vi "Edit Line.vi"(8 "error in":errorcluster, 10 "Line Name":string, 11 "References":T1) -> (0 "error out":errorcluster, 2 "change?":bool)   [LabVIEW 2013, in "shared memory editor node.lvclass"]
doc: "This VI edits the properties of a line. It will unlink channels and tags and create new links to channels and tags."
uses:
  shared memory editor node.lvclass
  <vilib>/NI/DCAF/Tag Editor Core/Table API/Table Manager/object ref.ctl
  <vilib>/NI/DCAF/Tag Editor Core/Configuration Editor/Classes/Engine Parent/Engine Parent Editor Node.lvclass
  <vilib>/NI/DCAF/Tag Editor Core/Configuration Editor/Classes/Module editor node/module editor node.lvclass
  module/configuration/shared memory configuration.lvclass
  module/configuration/shared memory configuration.lvclass/shared memory configuration.ctl
  <vilib>/NI/Configuration Framework/serializable configuration/NISE_CEF_serializable configuration.lvclass/NISE_CEF_serializable configuration.ctl
  <vilib>/Utility/LVClass/Get LV Class Name.vi
  <vilib>/NI/Configuration Framework/error generator/NISE_error generator.vi
  <vilib>/NI/Configuration Framework/serializable configuration/NISE_CEF_serializable configuration.lvclass
  <vilib>/NI/DCAF/Tag Editor Core/Table API/Table Manager/Table Manager.lvclass
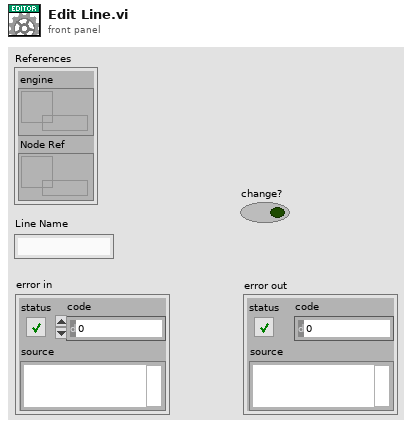
[diagram p1: front panel]
types:
  T1 = typedef "Table Manager.lvlib/Table Manager.lvclass/object ref.ctl" = cluster{"engine":refnum<data-value>, "Node Ref":refnum<data-value>}
  T2 = typedef "shared memory configuration.lvclass/Line.ctl" = cluster{"name":string, "data type":T3, "channel":refnum<class "TBM channel.lvclass">}
  T3 = typedef "tag bus.lvlib/tag descriptor.lvclass/Data Type.ctl" = enum16{"Double", "Single", "I64", "I32", "I16", "I8", "U64", "U32", "U16", "U8", "Boolean", "String", "Array of Double", "Array of Single", "Array of I64", "Array of I32", "Array of I16", "Array of I8", "Array of U64", "Array of U32", "Array of U16", "Array of U8", "Array of Boolean", "Array of String"}
  T4 = typedef "shared memory editor node.lvclass/Mappings.ctl" = cluster{"Line":T2, "Maps":T5[]}
  T5 = typedef "shared memory editor node.lvclass/Map.ctl" = cluster{"channel":refnum<class "TBM channel.lvclass">, "tag name":string}
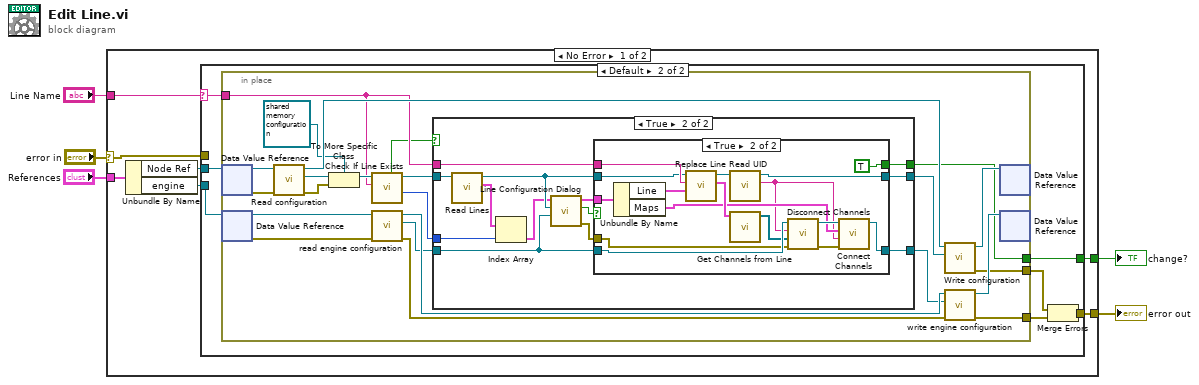
[diagram p0: block diagram]
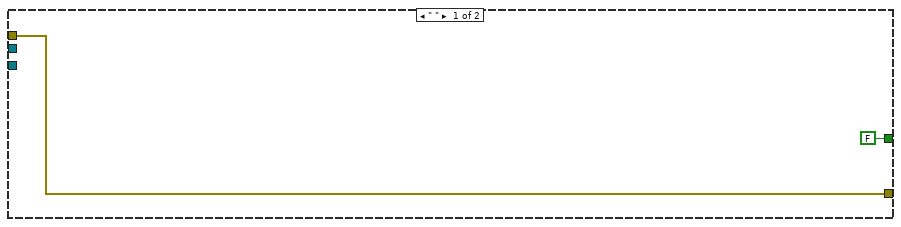
[diagram p2: hidden frame]
diagram:
  n1 = case shown="No Error" "error in" {
    selector: "error in" -> [w6 w78]
    tunnel: "References" -> [w10 _]
    tunnel: "Line Name" -> [w7 _]
    tunnel: [w9 w78] -> w2
    tunnel: [w8 _] -> w1
    frame No Error {
      n2 = Unbundle By Name(w10) -> ("Node Ref"=w12:refnum<data-value>, "engine"=w11:refnum<data-value>)
      n3 = case shown="Default" w7 {
        selector: w7 -> [_ w15]
        tunnel: w12 -> [_ w21]
        tunnel: w11 -> [_ w20]
        tunnel: [w13 w17] -> w9
        tunnel: [FALSE ("change?") w16] -> w8
        tunnel: w6 -> [w13 _]
        frame " " {
        }
        frame Default {
          n4 = in-place {
            in-place-border: [w25] -> w19
            in-place-border: [w41] -> w18
            in-place-border: [w24] -> w16
            in-place-border: w15 -> [w30]
            n5 = in-place-dvr #1(w21) -> (w37:refnum<class "module editor node.lvclass">, w31:errorcluster)
            n6 = in-place-dvr #2(w20) -> (w44:refnum<class "Engine Parent Editor Node.lvclass">, w43:errorcluster)
            n7 = call-dynamic "Read configuration.vi"("error in"=w31, "NISE_CEF_serializable node in"=w37) -> ("error out"=w34:errorcluster, "configuration"=w35:refnum<class "NISE_CEF_serializable configuration.lvclass">, "NISE_CEF_serializable node out"=w36:refnum<class "module editor node.lvclass">)  [unwired: 7 in]
            n8 = To More Specific Class(target class=refnum<class "shared memory configuration.lvclass"> refnum ("tag bus configurable plugin module configuration"), reference=w35, error in=w34) -> (specific class reference=w32:refnum<class "shared memory configuration.lvclass">)  [unwired: 1 out]
            n9 = call-dynamic "Check If Line Exists.vi"("Name to Locate"=w30, "shared memory configuration in"=w32) -> ("Index"=w27:i32, "shared memory configuration out"=w28:refnum<class "shared memory configuration.lvclass">, "Found?"=w22:bool)  [unwired: 5 in, 2 out]
            n10 = call <vilib>:"read engine configuration.vi"("error in"=w43, "Engine Parent Editor Node in"=w44) -> ("error out"=w39:errorcluster, "engine configuration"=w26:refnum<class "engine configuration.lvclass">, "Engine Parent Editor Node out"=w40:refnum<class "Engine Parent Editor Node.lvclass">)  [unwired: 7 in]
            n11 = case shown="True" w22 {
              tunnel: w28 -> [w46 w57]
              tunnel: w26 -> [w45 w47]
              tunnel: w30 -> [_ w59]
              tunnel: [w46 w51] -> w29
              tunnel: w27 -> [_ w54]
              tunnel: [_ w49] -> w24
              tunnel: [w45 w48] -> w23
              frame False {
              }
              frame True {
                n12 = call "Read Lines.vi"("shared memory configuration in"=w57) -> ("Lines"=w55:T2[], "shared memory configuration out"=w56:refnum<class "shared memory configuration.lvclass">)  [unwired: 8 in, 1 out]
                n13 = Index Array(array=w55, index=w54) -> (element=w53:T2)
                n14 = call "Line Configuration Dialog.vi"("engine configuration in"=w47, "tag bus configurable plugin module configuration"=w56, "Line"=w53) -> ("error out"=w58:errorcluster, "changed"=w50:bool, "Mappings out"=w52:T4)  [unwired: 5 in, 1 out]
                n15 = case shown="True" w50 {
                  tunnel: w59 -> [_ w77]
                  tunnel: w47 -> [w60 w76]
                  tunnel: w58 -> [_ w75]
                  tunnel: w56 -> [w61 w71]
                  tunnel: w52 -> [_ w70]
                  tunnel: [w61 w68] -> w51
                  tunnel: [_ TRUE ("change?")] -> w49
                  tunnel: [w60 w62] -> w48
                  frame False {
                  }
                  frame True {
                    n16 = Unbundle By Name(w70) -> ("Line"=w69:T2, "Maps"=w65:T5[])
                    n17 = call "Replace Line.vi"("New Line"=w69, "Line Name"=w77, "shared memory configuration in"=w71) -> ("Old Line"=w73:T2, "shared memory configuration out"=w74:refnum<class "shared memory configuration.lvclass">)  [unwired: 6 in, 1 out]
                    n18 = call <vilib>:"Read UID.vi"("configuration in"=w74) -> ("instance id"=w64:string, "configuration out"=w68:refnum<class "shared memory configuration.lvclass">)  [unwired: 8 in, 1 out]
                    n19 = call "Get Channels from Line.vi"("Line"=w73) -> ("Channels"=w72:refnum<class "TBM channel.lvclass">[])  [unwired: 10 in]
                    n20 = call "Disconnect Channels.vi"("error in (no error)"=w75, "Deleted Channels"=w72, "instance id"=w64, "Engine Configuration in"=w76) -> ("error out"=w66:errorcluster, "Engine Configuration out"=w67:refnum<class "engine configuration.lvclass">)  [unwired: 6 in]
                    n21 = call "Connect Channels.vi"("error in (no error)"=w66, "instance id"=w64, "Maps"=w65, "Engine Configuration in"=w67) -> ("Engine Configuration out"=w62:refnum<class "engine configuration.lvclass">)  [unwired: 6 in, 1 out]
                  }
                }
              }
            }
            n22 = call-dynamic "Write configuration.vi"("configuration"=w29, "NISE_CEF_serializable node in"=w36) -> ("error out"=w25:errorcluster, "NISE_CEF_serializable node out"=w38:refnum<class "module editor node.lvclass">)  [unwired: 8 in]
            n23 = call <vilib>:"write engine configuration.vi"("error in"=w39, "engine configuration"=w23, "Engine Parent Editor Node in"=w40) -> ("error out"=w41:errorcluster, "Engine Parent Editor Node out"=w42:refnum<class "Engine Parent Editor Node.lvclass">)  [unwired: 7 in]
            n24 = in-place-dvr #1(w38) -> ()  [unwired: 2 out]
            n25 = in-place-dvr #2(w42) -> ()  [unwired: 2 out]
          }
          n26 = Merge Errors(w19, w18) -> (w17:errorcluster)
        }
      }
    }
    frame Error {
    }
  }
  "change?" <- w1
  "error out" <- w2
